vi "get_central_wav_and_fwhm.vi"(2 "Signal":dbl[](array[numeric]), 3 "Wavelenghs":dbl[](array[numeric])) -> (0 "FWHM":dbl, 1 "Central":dbl)   [LabVIEW 2018]
uses:
  <vilib>/Analysis/6fits.llb/Curve Fitting Criteria.ctl
  <vilib>/Analysis/NI_AALPro.lvlib
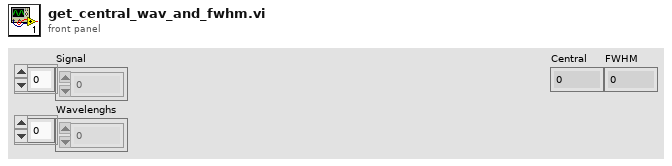
[diagram p1: front panel]
types:
  T1 = typedef "NI_AALPro.lvlib/Curve Fitting Criteria.ctl" = u16
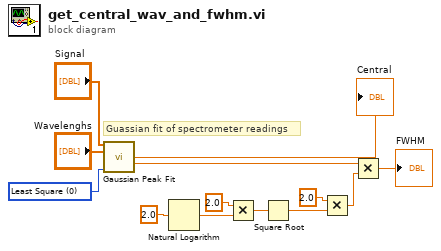
[diagram p0: block diagram]
diagram:
  w5 = T1 0 items=["Least Square", "Least Absolute Residual", "Bisquare"] ("method")
  # "Guassian fit of spectrometer readings"
  n1 = call <vilib>:"Gaussian Peak Fit.vi"("Y"="Signal", "X"="Wavelenghs", "method"=w5) -> ("center"=→"Central":dbl, "standard deviation"=w6:dbl)  [unwired: 6 in, 5 out]
  n2 = Natural Logarithm(1:2.0 ("x")) -> (0:w12:dbl)
  n3 = Multiply(x=2.0, y=w12) -> (x*y=w10:dbl)
  n4 = Square Root(x=w10) -> (sqrt(x)=w9:dbl)
  n5 = Multiply(x=2.0, y=w9) -> (x*y=w7:dbl)
  n6 = Multiply(x=w6, y=w7) -> (x*y=→"FWHM":dbl)
